vi "Configure Dialog.vi"(8 "error in (no error)":errorcluster, 11 "Message in":refnum<class "Message.lvclass">) -> (0 "error out":errorcluster, 2 "Ok?":bool, 3 "Message out":refnum<class "Message.lvclass">)   [LabVIEW 2014, in "Dialog PV Template.lvclass"]
uses:
  Dialog PV Template.lvclass
  <vilib>/ActorFramework/Message/Message.lvclass
panel:
  in  "Cancel Button":bool
  in  "OK Button":bool
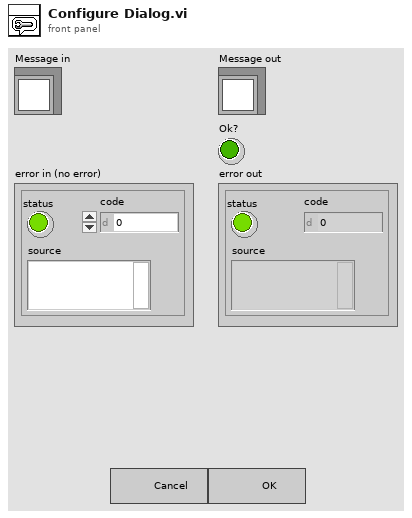
[diagram p1: front panel]
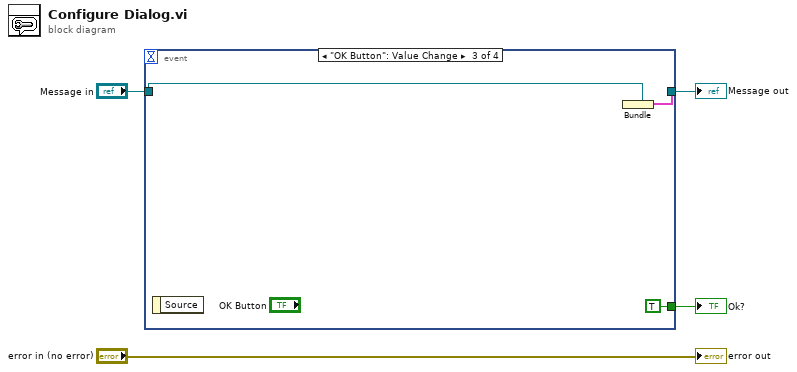
[diagram p0: block diagram]
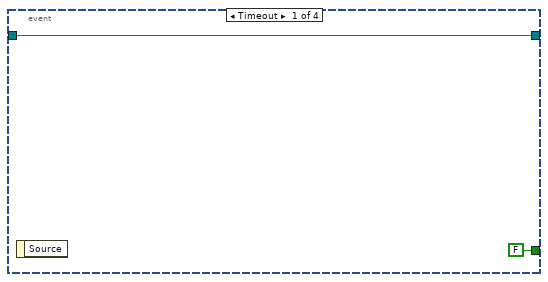
[diagram p2: hidden frame]
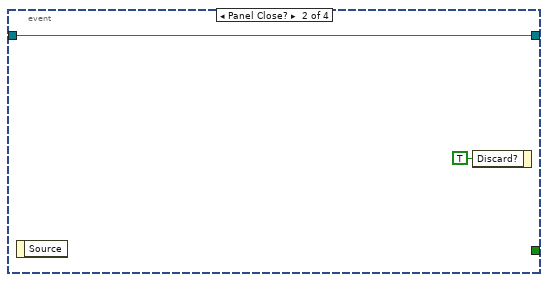
[diagram p3: hidden frame]
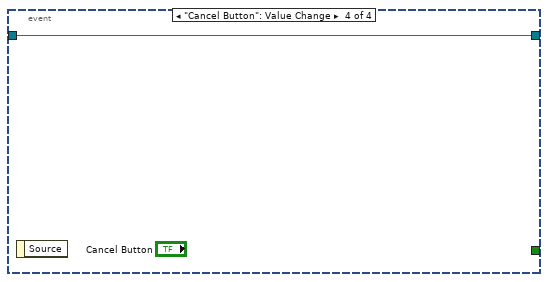
[diagram p4: hidden frame]
diagram:
  n1 = event shown="[2] \"OK Button\": Value Change" {
    selector: _ -> [_ _ _ _]
    dyn-events: _ -> [_ _ _ _]
    timeout: _ -> [_ _ _ _]
    tunnel: [w5 w7 w9 w12] -> w2
    tunnel: "Message in" -> [w5 w7 w11 w12]
    tunnel: [FALSE _ TRUE _] -> w3
    event Timeout {
      n2 = event-data() -> ()  [unwired: 1 in, 1 out]
    }
    event Panel Close? {
      n3 = event-data() -> ()  [unwired: 1 in, 1 out]
      n4 = event-data("Discard?"=TRUE) -> ()  [unwired: 1 in, 1 out]
    }
    event "OK Button": Value Change {
      n5 = event-data() -> ()  [unwired: 1 in, 1 out]
      n6 = Bundle ("Main-Bundler")(cluster=w11) -> (w9:cluster{void})  [unwired: 1 in]
    }
    event "Cancel Button": Value Change {
      n7 = event-data() -> ()  [unwired: 1 in, 1 out]
    }
  }
  "Ok?" <- w3
  "Message out" <- w2
  "error out" <- "error in (no error)"
